vi "triad_error.vi"(9 "Measured positions":T2 format="%#.1f", 10 "Measure transform":T1, 11 "Calibrated positions":T2 format="%#.1f") -> (2 "Residues":T2 format="%#.1f", 3 "RMS error":dbl)   [LabVIEW 2014]
uses:
  probe_calibration.ctl
  <vilib>/Analysis/Matrix/Datatypes/RealMatrix.ctl
  <vilib>/Analysis/baseanly.llb/A x Vector.vi
  <vilib>/Analysis/NI_AALBase.lvlib
  <vilib>/Analysis/Matrix/NI_Matrix.lvlib
panel:
  # "When the measured positions are transformed they should map onto the calibrated positions.  Any mismatch is error in the calibration.     We call this triad error because it amounts to disagreement over the shape of the triad of measurements (the LED triangle or fiducials.)"
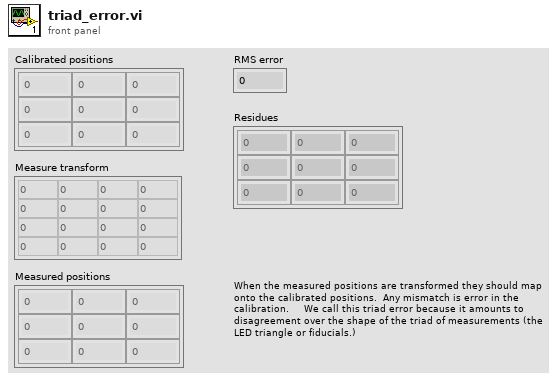
[diagram p1: front panel]
types:
  T1 = typedef "NI_Matrix.lvlib/RealMatrix.ctl" = dbl[][]
  T2 = typedef "probe_calibration.ctl" = sgl[][]
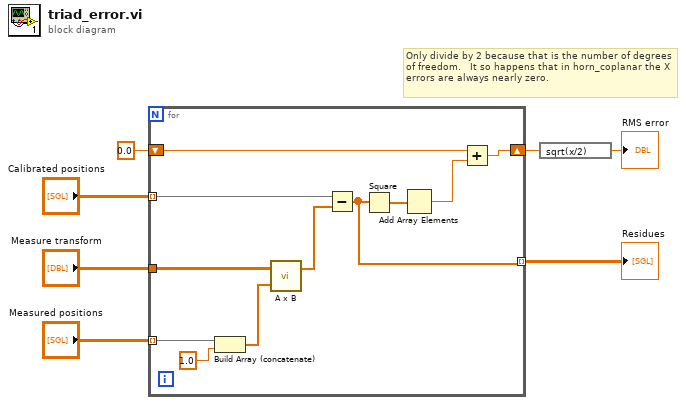
[diagram p0: block diagram]
diagram:
  # "Only divide by 2 because that is the number of degrees of freedom.   It so happens that in horn_coplanar the X errors are always nearly zero."
  n1 = for {
    tunnel: "Measured positions" -> [w8] mode=indexing
    tunnel: "Measure transform" -> [w17]
    tunnel: "Calibrated positions" -> [w15] mode=indexing
    shift-right: [w12] -> w7
    shift-left: 0.0 ("length") -> [w10]
    tunnel: [w9] -> w4 mode=indexing
    n2 = Build Array (concatenate)(w8, sgl 1.0) -> (w16:sgl[])
    n3 = call-poly <vilib>:"A x B.vi"("Vector"=w16, "A"=w17) -> ("A x Vector"=w14:dbl[])  [unwired: 1 out]
    n4 = Subtract(x=w15, y=w14) -> (x-y=w9:dbl[])
    n5 = Square(x=w9) -> (x^2=w13:dbl[])
    n6 = Add Array Elements(numeric array=w13) -> (sum=w11:dbl)
    n7 = Add(x=w10, y=w11) -> (x+y=w12:dbl)
  }
  "Residues" <- w4
  n8 = expression code="sqrt(x/2)"(w7) -> (→"RMS error":dbl)
